vi "robot_init.vi"(10 "Remote port":u16=30002, 11 "IP-address":string="192.168.0.1") -> (0 "error out":errorcluster, 3 "connection ID":refnum<k5>)   [LabVIEW 2022 SP3]
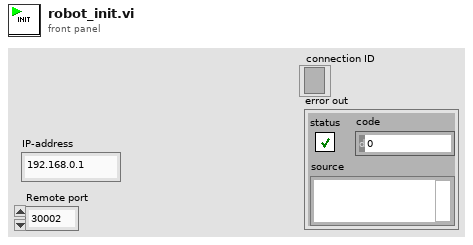
[diagram p1: front panel]
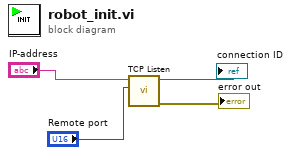
[diagram p0: block diagram]
diagram:
  n1 = call <vilib>:"TCP Listen.vi"("port"="Remote port", "service name"="IP-address") -> ("error out"=→"error out":errorcluster, "connection ID"=→"connection ID":refnum<k5>)  [unwired: 5 in, 3 out]
